vi "Test DAQ Hardware API.vi"() -> ()   [LabVIEW 2016]
doc: "DAQ Hardware API Tester."
uses:
  DAQ Hardware.lvlib
  <vilib>/Utility/error.llb/DialogType.ctl
  <vilib>/Utility/miscctls.llb/LVPointTypeDef.ctl
  User Interface/AI Channel Setting.ctl
  Timing AI DAQ Setting.ctl
  AO Channel Setting.ctl
  DI Channel Setting.ctl
  DO Channel Setting.ctl
  AO Name.ctl
panel:
  in  "REQ Log Data":bool
  in  "Value":dbl
  in  "AO Name":T1
  in  "REQ Retry DI":bool
  in  "REQ Wakeup_helper_loop_DI":bool
  in  "REQ Retry AI":bool
  in  "REQ Wakeup_Helper_loop_AI":bool
  in  "Automatic":bool=TRUE
  out "AI Data":dbl[][](array[numeric])
  out "DI":bool[](array[boolean])
  in  "REQ Acquire DI":bool
  in  "DO Channel Setting":T2={"DO Channel"=["6363/port1/line0", "6363/port1/line1", "6363/port1/line2", "6363/port1/line3"]}
  in  "DI Channel Setting":T3={"DI Channel"=["6363/port0/line0", "6363/port0/line1", "6363/port0/line2", "6363/port0/line3"]}
  in  "AO Channel Setting":T4={"AO Channel name"=["6363/ao0", "6363/ao1", "6363/ao2", "6363/ao3"], "output terminal configuration"=enum."RSE", "minimum value"=-10.0, "maximum value"=10.0, "units"=enum."Volts", "name to assign"=[]} {"maximum value" format="%0.2f"; "minimum value" format="%0.2f"}
  in  "Timing Parameter":T5={"rate"=5000.0, "samples per channel"=1000, "sample mode"=10123} {"sample mode" items=["Finite Samples"=10178, "Continuous Samples"=10123, "Hardware Timed Single Point"=12522]; "samples per channel" min=100; "rate" min=1000.0 format="%0.2f"}
  in  "REQ Update Sample Rate":bool
  in  "AI Setting":T6={"Physical Channel"=["6363/ai0", "6363/ai1", "6363/ai3"], "Name to assign"=["AI 0", "AI 1", "AI 3"], "minimum value"=0.0, "maximum value"=10.0, "custom scale name"="", "rate"=5000.0, "samples per channel"=1000, "input terminal configuration"=2, "units"=0, "sample mode"=2} {"sample mode" items=["Finite Samples"=10178, "Continuous Samples"=10123, "Hardware Timed Single Point"=12522]; "units" items=["Volts"=10348, "From Custom Scale"=10065]; "input terminal configuration" items=["Finite Samples", "Continuous Samples", "Hardware Timed Single Point"]; "rate" format="%#_13g"; "maximum value" format="%#_13g"; "minimum value" format="%#_13g"}
  in  "Value":dbl[](array[numeric])
  in  "REQ Write AO":bool
  in  "REQ Close Ref":bool
  in  "REQ Acquire AI":bool
  out "Connect?":bool
  out "Connect?":bool
  out "Connect?":bool
  in  "DO Value":bool[](array[boolean])
  in  "REQ Write DO":bool
  in  "REQ Initialize DO":bool
  in  "REQ Initialize DI":bool
  in  "REQ Initialize AO":bool
  out "Connect?":bool
  in  "DAQ Type":enum16{"Hardware", "Simulation"}(ring)
  in  "REQ Initialize AI":bool
  in  "Show Diagram on Init":bool
  in  "Show Block Diagram":bool
  in  "Stop Module":bool
  in  "Start Module":bool
  in  "Hide Module Panel":bool
  in  "Show Module Panel":bool
  out "Status":string
  out "Module Running?":bool
  # "This VI tests the API for the Module."
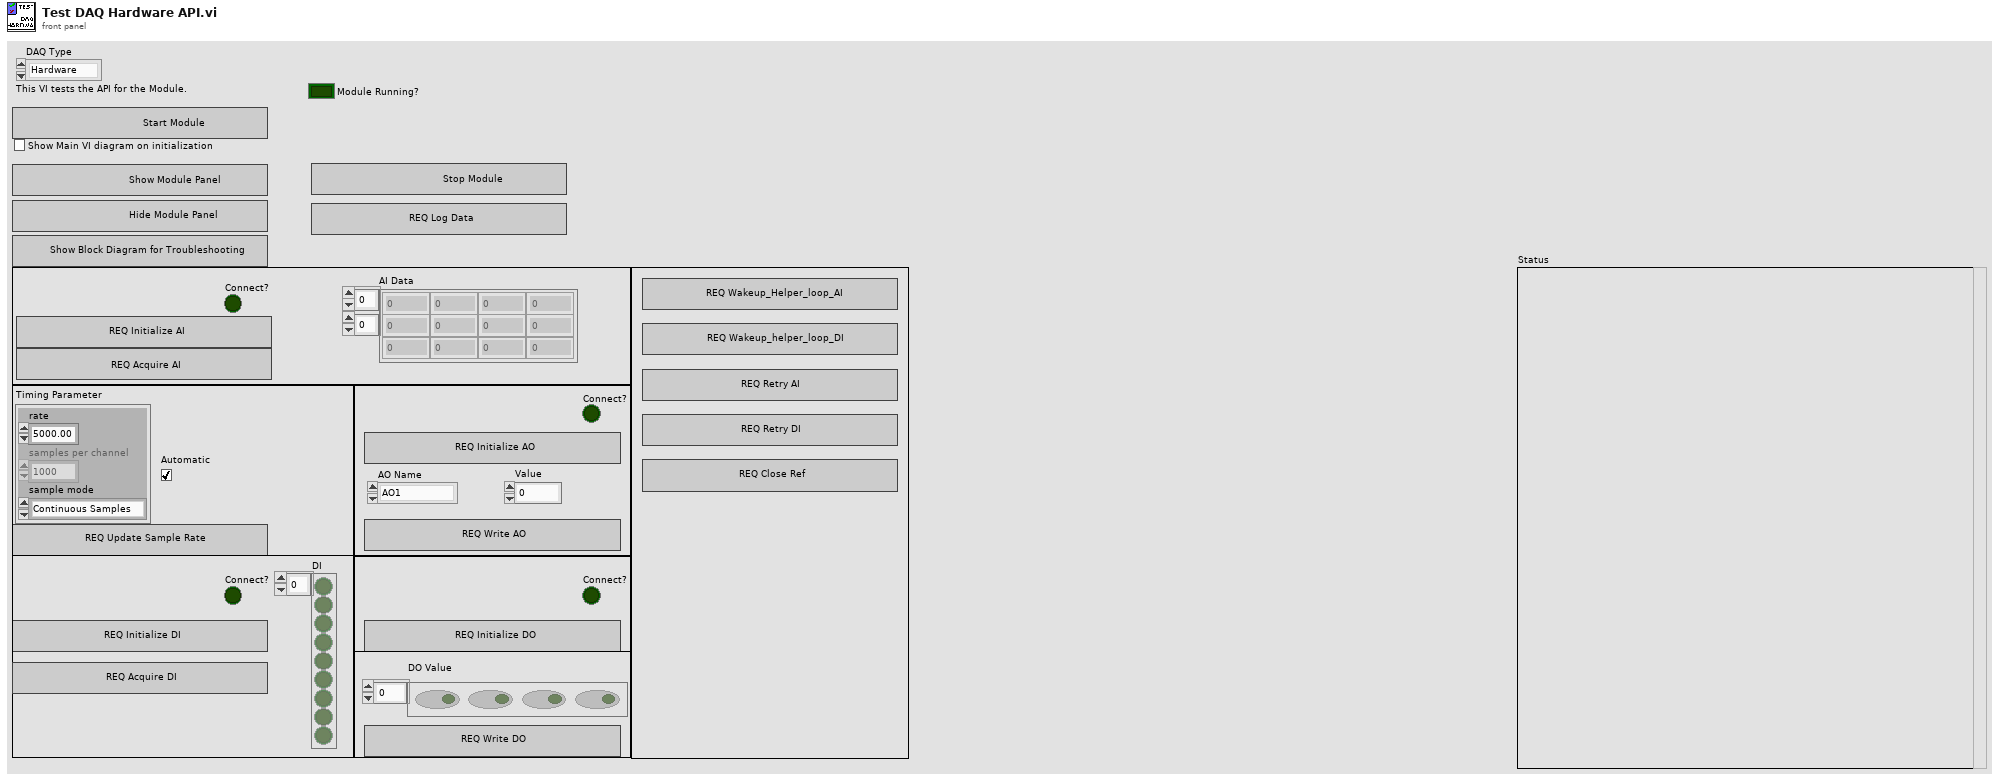
[diagram p1: front panel]
types:
  T1 = typedef "DAQ Hardware.lvlib/AO Name.ctl" = enum16{"AO1", "AO2", "AO3", "AO4"}
  T2 = typedef "DAQ Hardware.lvlib/DO Channel Setting.ctl" = cluster{"DO Channel":string[]}
  T3 = typedef "DAQ Hardware.lvlib/DI Channel Setting.ctl" = cluster{"DI Channel":string[]}
  T4 = typedef "DAQ Hardware.lvlib/AO Channel Setting.ctl" = cluster{"AO Channel name":string[], "output terminal configuration":enum16{"RSE", "NRSE", "Differential"}, "minimum value":dbl, "maximum value":dbl, "units":enum16{"Volts"}, "name to assign":string[]}
  T5 = typedef "DAQ Hardware.lvlib/Timing AI DAQ Setting.ctl" = cluster{"rate":dbl, "samples per channel":i32, "sample mode":i32}
  T6 = typedef "DAQ Hardware.lvlib/AI Channel Setting.ctl" = cluster{"Physical Channel":string[], "Name to assign":string[], "minimum value":dbl, "maximum value":dbl, "custom scale name":string, "rate":dbl, "samples per channel":i32, "input terminal configuration":i32, "units":i32, "sample mode":i32}
  T7 = typedef "LVPointTypeDef.ctl" = cluster{"Horizontal":i16, "Vertical":i16}
  T8 = typedef "DAQ Hardware.lvlib/Broadcast Events--cluster.ctl" = cluster{"Module Did Init":refnum<user-event>, "Status Updated":refnum<user-event>, "Error Reported":refnum<user-event>, "Module Did Stop":refnum<user-event>, "Update Module Execution Status":refnum<user-event>, "REQ Broadcast DI":refnum<user-event>, "REQ Broad AI":refnum<user-event>}
  T9 = enum8{"Enabled", "Disabled", "Disabled and Grayed Out"}
  T10 = typedef "DialogType.ctl" = u16
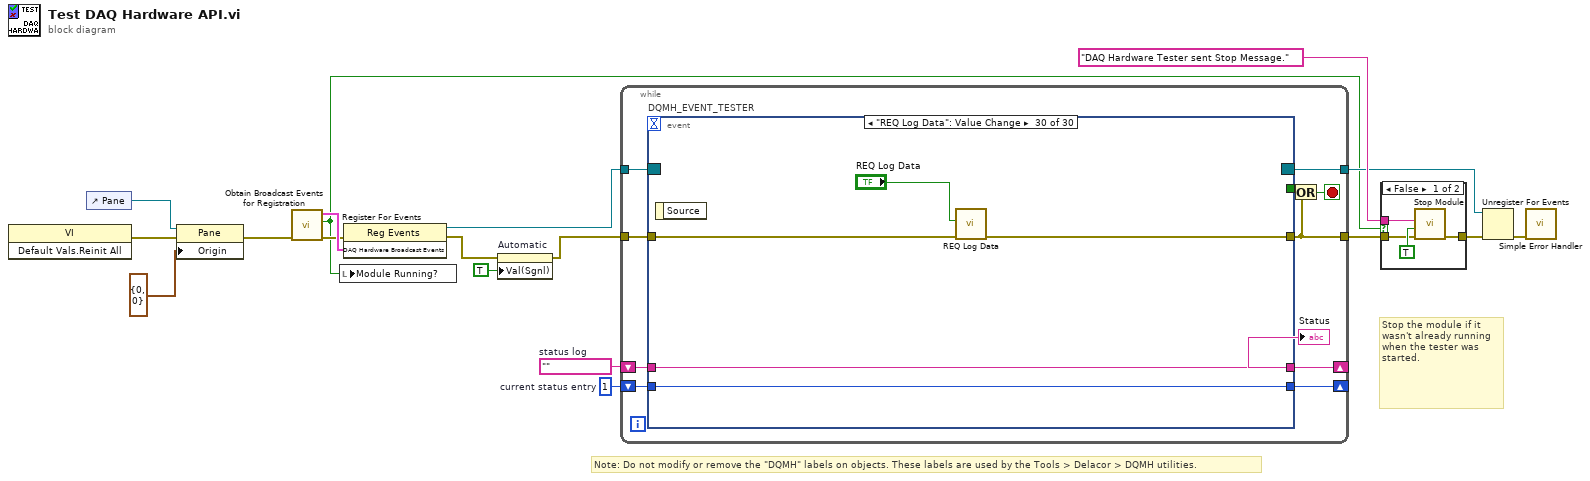
[diagram p0: block diagram]
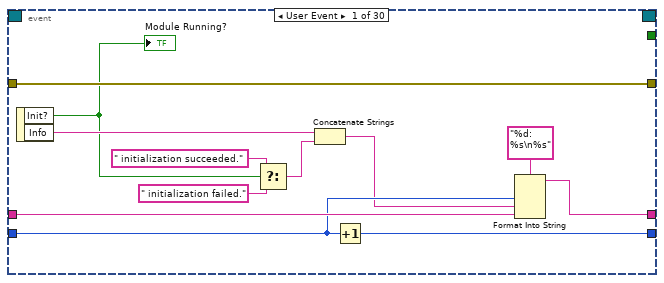
[diagram p3: hidden frame]
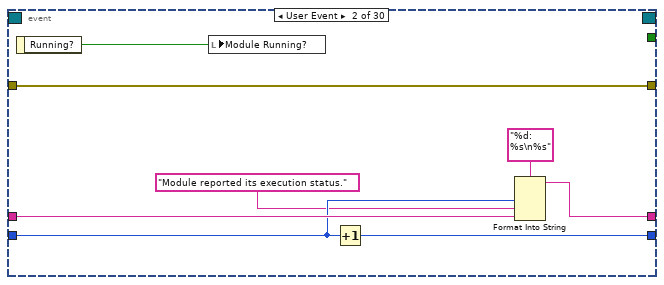
[diagram p4: hidden frame]
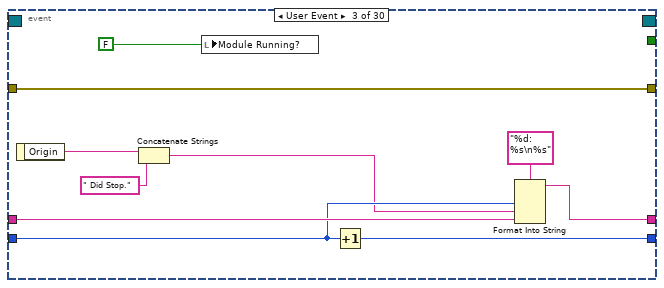
[diagram p5: hidden frame]
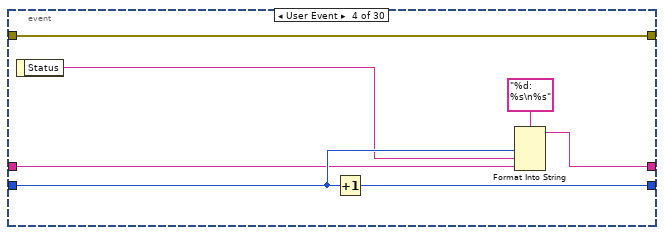
[diagram p6: hidden frame]
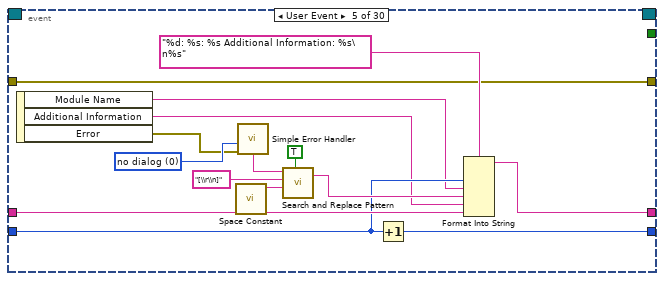
[diagram p7: hidden frame]
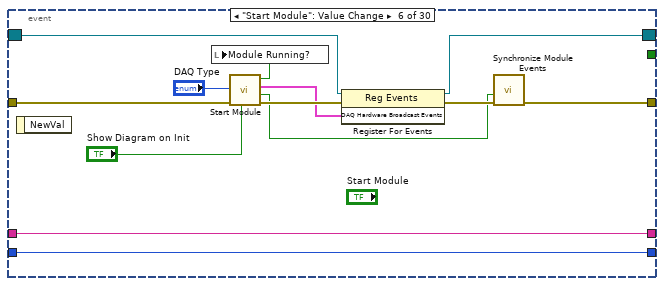
[diagram p8: hidden frame]
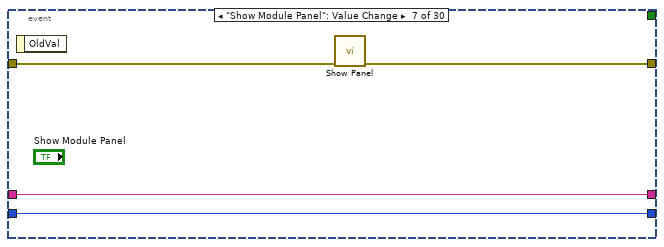
[diagram p9: hidden frame]
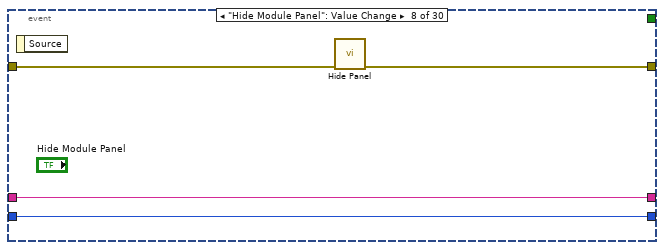
[diagram p10: hidden frame]
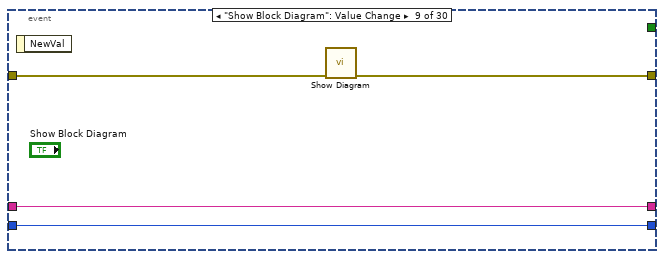
[diagram p11: hidden frame]
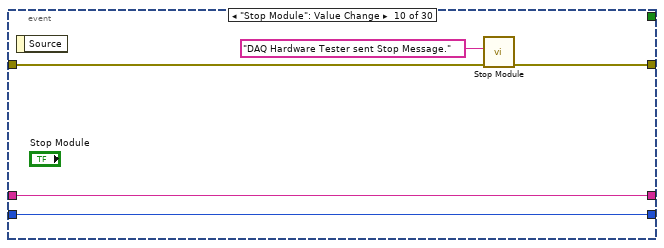
[diagram p12: hidden frame]
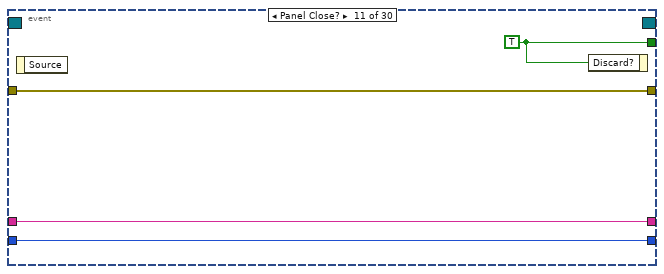
[diagram p13: hidden frame]
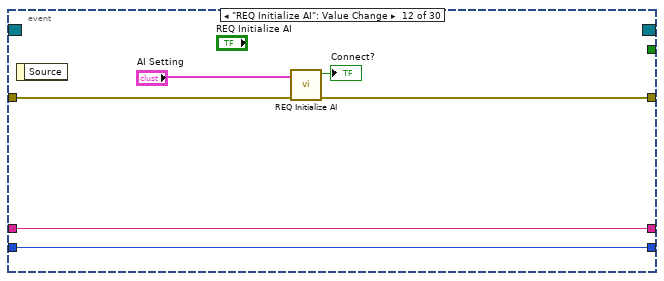
[diagram p14: hidden frame]
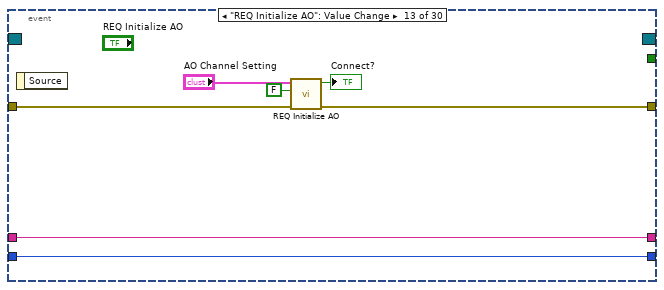
[diagram p15: hidden frame]
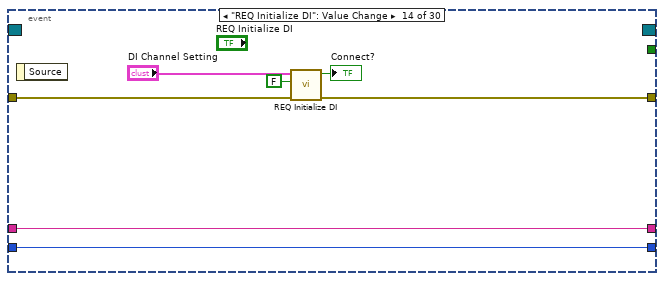
[diagram p16: hidden frame]
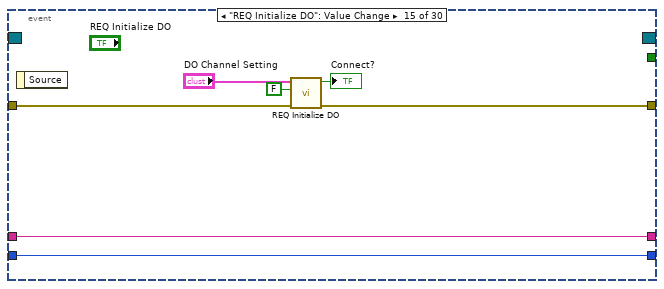
[diagram p17: hidden frame]
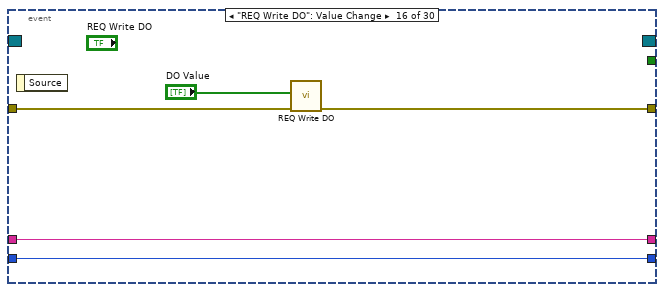
[diagram p18: hidden frame]
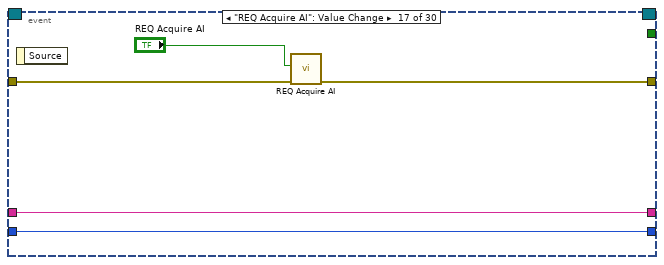
[diagram p19: hidden frame]
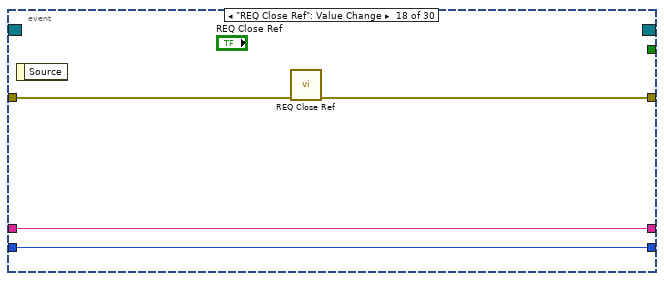
[diagram p20: hidden frame]
diagram:
  w15 = 1  # current status entry
  w16 = ""  # status log
  # "Stop the module if it wasn't already running when the tester was started."
  # "Note: Do not modify or remove the \"DQMH\" labels on objects. These labels are used by the Tools > Delacor > DQMH utilities."
  n1 = invoke class="VI" method="Default Vals.Reinit All"() -> (error out=w3:errorcluster)  [unwired: 3 in, 2 out]
  n2 = control-ref of="Pane"() -> (w4:refnum<vi>)
  n3 = property class="Pane"(reference=w4, error in=w3, "Origin"=T7 {"Horizontal"=0, "Vertical"=0}) -> (error out=w2:errorcluster)  [unwired: 1 out]
  n4 = call "Obtain Broadcast Events for Registration.vi"("error in"=w2) -> ("error out"=w11:errorcluster, "Already running?"=w10:bool, "DAQ Hardware Broadcast Events"=w14:T8)  [unwired: 8 in]
  n5 = local write "Module Running?"(w10) -> ()
  n6 = register-events(error in=w11, w14) -> (reference out=w13:refnum<event-registration>, error out=w7:errorcluster)  [unwired: 1 in]
  n7 = property on="Automatic" class="Bool (strict)"(error in=w7, "Val(Sgnl)"=TRUE ("Value (Signaling)")) -> (error out=w6:errorcluster)  [unwired: 1 in, 1 out]
  n8 = while {
    tunnel: w13 -> [w28]
    tunnel: [w19] -> w9
    shift-right: [w23] -> _
    shift-left: w16 -> [w25]
    shift-right: [w24] -> _
    shift-left: w15 -> [w26]
    tunnel: w6 -> [w21]
    tunnel: [w20] -> w12
    stop <- w22 stop-if-true
    n9 = event "DQMH_EVENT_TESTER" shown="[29] \"REQ Log Data\": Value Change" {
      selector: w28 -> [_ _ _ _ _ w87 _ _ _ _ _ _ _ _ _ _ _ _ _ _ _ _ _ _ _ _ _ _ _ _]
      dyn-events: [_ _ _ _ _ w86 _ _ _ _ _ _ _ _ _ _ _ _ _ _ _ _ _ _ _ _ _ _ _ _] -> w20
      timeout: _ -> [_ _ _ _ _ _ _ _ _ _ _ _ _ _ _ _ _ _ _ _ _ _ _ _ _ _ _ _ _ _]
      tunnel: [_ _ _ _ _ _ _ _ _ _ w114 _ _ _ _ _ _ _ _ _ _ _ _ _ _ _ _ _ _ _] -> w27
      tunnel: [w40 w42 w49 w59 w69 w85 w97 w101 w102 w108 w111 w117 w124 w131 w138 w143 w148 w152 w160 w165 w176 w177 w192 w194 w205 w208 w212 w217 w221 w226] -> w19
      tunnel: w26 -> [w37 w46 w56 w62 w72 w90 w95 w99 w103 w109 w112 w118 w125 w132 w139 w144 w149 w153 w161 w166 w174 w183 w187 w195 w200 w209 w213 w218 w222 w227]
      tunnel: w25 -> [w38 w47 w57 w61 w73 w91 w96 w100 w104 w110 w113 w119 w126 w133 w140 w145 w150 w154 w162 w167 w175 w184 w185 w196 w201 w210 w214 w219 w223 w228]
      tunnel: [w35 w44 w54 w63 w71 w91 w96 w100 w104 w110 w113 w119 w126 w133 w140 w145 w150 w154 w162 w167 w175 w184 w185 w196 w201 w210 w214 w219 w223 w228] -> w23
      tunnel: [w36 w45 w55 w65 w70 w90 w95 w99 w103 w109 w112 w118 w125 w132 w139 w144 w149 w153 w161 w166 w174 w183 w187 w195 w200 w209 w213 w218 w222 w227] -> w24
      tunnel: w21 -> [w40 w42 w49 w59 w69 w84 w94 w98 w105 w106 w111 w120 w127 w134 w141 w146 w151 w155 w163 w168 w176 w178 w192 w197 w205 w211 w215 w220 w224 w229]
      event User Event {
        n10 = event-data() -> ("Init?"=w32:bool, "Info"=w34:string)  [unwired: 1 in]
        "Module Running?" <- w32
        n11 = Select(t=" initialization succeeded.", s=w32, f=" initialization failed.") -> (s? t:f=w29:string)
        n12 = Concatenate Strings(w34, w29) -> (w33:string)
        n13 = Increment(x=w37) -> (x+1=w36:i32)
        n14 = Format Into String(format string="%d: %s\n%s", w37, w33, w38) -> (resulting string=w35:string)  [unwired: 2 in, 1 out]
      }
      event User Event {
        n15 = event-data() -> ("Running?"=w41:bool)  [unwired: 1 in]
        n16 = local write "Module Running?"(w41) -> ()
        n17 = Increment(x=w46) -> (x+1=w45:i32)
        n18 = Format Into String(format string="%d: %s\n%s", w46, "Module reported its execution status.", w47) -> (resulting string=w44:string)  [unwired: 2 in, 1 out]
      }
      event User Event {
        n19 = event-data() -> ("Origin"=w53:string)  [unwired: 1 in]
        n20 = Concatenate Strings(w53, " Did Stop.") -> (w52:string)
        n21 = local write "Module Running?"(FALSE ("Module Did Init?")) -> ()
        n22 = Increment(x=w56) -> (x+1=w55:i32)
        n23 = Format Into String(format string="%d: %s\n%s", w56, w52, w57) -> (resulting string=w54:string)  [unwired: 2 in, 1 out]
      }
      event User Event {
        n24 = event-data() -> ("Status"=w60:string)  [unwired: 1 in]
        n25 = Increment(x=w62) -> (x+1=w65:i32)
        n26 = Format Into String(format string="%d: %s\n%s", w62, w60, w61) -> (resulting string=w63:string)  [unwired: 2 in, 1 out]
      }
      event User Event {
        w74 = T10 0 items=["no dialog", "OK message", "continue or stop message", "OK message + warnings", "continue/stop + warnings"] ("type of dialog (OK msg:1)")
        n27 = event-data() -> ("Module Name"=w68:string, "Additional Information"=w67:string, "Error"=w66:errorcluster)  [unwired: 1 in]
        n28 = call <vilib>:"Space Constant.vi"() -> ("String"=w78:string)
        n29 = call <vilib>:"Simple Error Handler.vi"("type of dialog (OK msg:1)"=w74, "error in (no error)"=w66) -> ("message"=w75:string)  [unwired: 3 in, 4 out]
        n30 = call <vilib>:"Search and Replace Pattern.vi"("string"=w75, "regular expression (\"\")"="[\\r\\n]" ("regular expression (\"\")"), "replace string (\"\")"=w78, "replace all? (F)"=TRUE ("replace all CR/LF with spaces")) -> ("result string"=w76:string)  [unwired: 1 in, 1 out]
        n31 = Increment(x=w72) -> (x+1=w70:i32)
        n32 = Format Into String(format string="%d: %s: %s Additional Information: %s\n%s", w72, w68, w76, w67, w73) -> (resulting string=w71:string)  [unwired: 2 in, 1 out]
      }
      event "Start Module": Value Change {
        n33 = event-data() -> ()  [unwired: 1 in, 1 out]
        n34 = call "Start Module.vi"("Show Main VI Diagram on Init (F)"="Show Diagram on Init", "error in"=w84, "DAQ Type"="DAQ Type") -> ("error out"=w92:errorcluster, "Wait for Event Sync?"=w89:bool, "DAQ Hardware Broadcast Events"=w88:T8, "Module Was Already Running?"=w83:bool)  [unwired: 5 in]
        n35 = local write "Module Running?"(w83) -> ()
        n36 = register-events(reference=w87, error in=w92, w88) -> (reference out=w86:refnum<event-registration>, error out=w93:errorcluster)
        n37 = call "Synchronize Module Events.vi"("error in"=w93, "Wait for Event Sync?"=w89) -> ("error out"=w85:errorcluster)  [unwired: 9 in]
      }
      event "Show Module Panel": Value Change {
        n38 = event-data() -> ()  [unwired: 1 in, 1 out]
        n39 = call "Show Panel.vi"("error in (no error)"=w94) -> ("error out"=w97:errorcluster)  [unwired: 10 in]
      }
      event "Hide Module Panel": Value Change {
        n40 = event-data() -> ()  [unwired: 1 in, 1 out]
        n41 = call "Hide Panel.vi"("error in (no error)"=w98) -> ("error out"=w101:errorcluster)  [unwired: 10 in]
      }
      event "Show Block Diagram": Value Change {
        n42 = event-data() -> ()  [unwired: 1 in, 1 out]
        n43 = call "Show Diagram.vi"("error in (no error)"=w105) -> ("error out"=w102:errorcluster)  [unwired: 10 in]
      }
      event "Stop Module": Value Change {
        n44 = event-data() -> ()  [unwired: 1 in, 1 out]
        n45 = call "Stop Module.vi"("error in"=w106, "Origin"="DAQ Hardware Tester sent Stop Message.") -> ("error out"=w108:errorcluster)  [unwired: 9 in]
      }
      event Panel Close? {
        w114 = TRUE ("Discard?")
        n46 = event-data() -> ()  [unwired: 1 in, 1 out]
        n47 = event-data("Discard?"=w114) -> ()  [unwired: 1 in, 1 out]
      }
      event "REQ Initialize AI": Value Change {
        n48 = event-data() -> ()  [unwired: 1 in, 1 out]
        n49 = call "REQ Initialize AI.vi"("error in"=w120, "AI Setting"="AI Setting") -> ("error out"=w117:errorcluster, "Connect?"=→"Connect?":bool)  [unwired: 7 in, 1 out]
      }
      event "REQ Initialize AO": Value Change {
        n50 = event-data() -> ()  [unwired: 1 in, 1 out]
        n51 = call "REQ Initialize AO.vi"("error in"=w127, "Boolean"=FALSE, "AO Channel Setting"="AO Channel Setting") -> ("error out"=w124:errorcluster, "Connect?"=→"Connect?":bool)  [unwired: 6 in, 1 out]
      }
      event "REQ Initialize DI": Value Change {
        n52 = event-data() -> ()  [unwired: 1 in, 1 out]
        n53 = call "REQ Initialize DI.vi"("error in"=w134, "Boolean"=FALSE, "DI Channel Setting"="DI Channel Setting") -> ("error out"=w131:errorcluster, "Connect?"=→"Connect?":bool)  [unwired: 6 in, 1 out]
      }
      event "REQ Initialize DO": Value Change {
        n54 = event-data() -> ()  [unwired: 1 in, 1 out]
        n55 = call "REQ Initialize DO.vi"("error in"=w141, "Boolean"=FALSE, "DO Channel Setting"="DO Channel Setting") -> ("error out"=w138:errorcluster, "Connect?"=→"Connect?":bool)  [unwired: 6 in, 1 out]
      }
      event "REQ Write DO": Value Change {
        n56 = event-data() -> ()  [unwired: 1 in, 1 out]
        n57 = call "REQ Write DO.vi"("error in"=w146, "DO Value"="DO Value") -> ("error out"=w143:errorcluster)  [unwired: 9 in]
      }
      event "REQ Acquire AI": Value Change {
        n58 = event-data() -> ()  [unwired: 1 in, 1 out]
        n59 = call "REQ Acquire AI.vi"("error in"=w151, "Acquire AI"="REQ Acquire AI") -> ("error out"=w148:errorcluster)  [unwired: 9 in]
      }
      event "REQ Close Ref": Value Change {
        n60 = event-data() -> ()  [unwired: 1 in, 1 out]
        n61 = call "REQ Close Ref.vi"("error in"=w155) -> ("error out"=w152:errorcluster)  [unwired: 10 in]
      }
      event "REQ Write AO": Value Change {
        n62 = event-data() -> ()  [unwired: 1 in, 1 out]
        n63 = Replace Array Subset(array=dbl[] [0.0, 0.0, 0.0, 0.0], new element="Value", index="AO Name") -> ()  [unwired: 1 out]
        n64 = call "REQ Write AO.vi"("error in"=w163, 9:"Value"="Value", 10:"Value"="Value", "AO Name"="AO Name") -> ("error out"=w160:errorcluster)  [unwired: 7 in]
      }
      event "REQ Update Sample Rate": Value Change {
        n65 = event-data() -> ()  [unwired: 1 in, 1 out]
        n66 = call "REQ Update Sample Rate.vi"("error in"=w168, "Timing Parameter"="Timing Parameter") -> ("error out"=w165:errorcluster)  [unwired: 9 in]
      }
      event Value Change {
        n67 = event-data() -> ("NewVal"=w172:dbl)  [unwired: 1 in]
        n68 = Divide(x=w172, y=10.0) -> (x/y=w170:dbl)
        n69 = local read "Timing Parameter"() -> (w171:T5)
        n70 = Bundle By Name(cluster=w171, "samples per channel"=w170) -> (w169:T5)
        n71 = local write "Timing Parameter"(w169) -> ()
      }
      event "Automatic": Value Change {
        n72 = event-data() -> ()  [unwired: 1 in, 1 out]
        n73 = Select(t=T9."Disabled and Grayed Out" ("Disabled"), s="Automatic", f=T9."Enabled" ("Disabled")) -> (s? t:f=w179:T9)
        n74 = property on="samples per channel" class="DigNum (strict)"(error in=w178, "DisabledEnum"=w179) -> (error out=w177:errorcluster)  [unwired: 1 in, 1 out]
      }
      event User Event {
        n75 = event-data() -> ("DI"=→"DI":bool[])  [unwired: 1 in, 1 out]
        n76 = Format Into String(format string="Response Received - %s", "" ("input 1")) -> (resulting string=w189:string)  [unwired: 2 in, 1 out]
        n77 = Increment(x=w187) -> ()  [unwired: 1 out]
        n78 = Format Into String(format string="%d: %s\n%s", w187, w189, w185) -> ()  [unwired: 2 in, 2 out]
      }
      event "REQ Acquire DI": Value Change {
        n79 = event-data() -> ()  [unwired: 1 in, 1 out]
        n80 = call "REQ Acquire DI.vi"("error in"=w197, "Acq DI"="REQ Acquire DI") -> ("error out"=w194:errorcluster)  [unwired: 9 in]
      }
      event User Event {
        n81 = event-data() -> ("AI Data"=→"AI Data":dbl[][])  [unwired: 1 in, 4 out]
        n82 = Format Into String(format string="Response Received - %s", "" ("input 1")) -> (resulting string=w202:string)  [unwired: 2 in, 1 out]
        n83 = Increment(x=w200) -> ()  [unwired: 1 out]
        n84 = Format Into String(format string="%d: %s\n%s", w200, w202, w201) -> ()  [unwired: 2 in, 2 out]
      }
      event "REQ Wakeup_Helper_loop_AI": Value Change {
        n85 = event-data() -> ()  [unwired: 1 in, 1 out]
        n86 = call "REQ Wakeup_Helper_loop_AI.vi"("error in"=w211, "Timeout"=-1, "Data"=variant) -> ("error out"=w208:errorcluster)  [unwired: 8 in]
      }
      event "REQ Retry AI": Value Change {
        n87 = event-data() -> ()  [unwired: 1 in, 1 out]
        n88 = call "REQ Retry AI.vi"("error in"=w215) -> ("error out"=w212:errorcluster)  [unwired: 10 in]
      }
      event "REQ Wakeup_helper_loop_DI": Value Change {
        # "#CodeNeeded\n1. Position the new \"REQ Wakeup_helper_loop_DI\" button appropriately on the front panel.\n2. Delete or edit this label when done."
        n89 = event-data() -> ()  [unwired: 1 in, 1 out]
        n90 = call "REQ Wakeup_helper_loop_DI.vi"("error in"=w220, "Data"=variant) -> ("error out"=w217:errorcluster)  [unwired: 9 in]
      }
      event "REQ Retry DI": Value Change {
        # "#CodeNeeded\n1. Position the new \"REQ Retry DI\" button appropriately on the front panel.\n2. Delete or edit this label when done."
        n91 = event-data() -> ()  [unwired: 1 in, 1 out]
        n92 = call "REQ Retry DI.vi"("error in"=w224) -> ("error out"=w221:errorcluster)  [unwired: 10 in]
      }
      event "REQ Log Data": Value Change {
        n93 = event-data() -> ()  [unwired: 1 in, 1 out]
        n94 = call "REQ Log Data.vi"("error in"=w229, "Log Data"="REQ Log Data") -> ("error out"=w226:errorcluster)  [unwired: 9 in]
      }
    }
    "Status" <- w23
    n95 = Or(x=w27, y=w19) -> (x .or. y?=w22:bool)
  }
  n96 = case shown="False" w10 {
    tunnel: [w233 w234] -> w18
    tunnel: "DAQ Hardware Tester sent Stop Message." ("Origin") -> [w232 _]
    tunnel: w9 -> [w230 w234]
    frame False {
      n97 = call "Stop Module.vi"("error in"=w230, "Wait for Module to Stop? (F)"=TRUE ("Wait for Module to stop?"), "Origin"=w232) -> ("error out"=w233:errorcluster)  [unwired: 8 in]
    }
    frame True {
    }
  }
  n98 = Unregister For Events(event registration refnum=w12, error in=w18) -> (error out=w8:errorcluster)
  n99 = call <vilib>:"Simple Error Handler.vi"("error in (no error)"=w8) -> ()  [unwired: 4 in, 5 out]
